vi "ReadI32Data.vi"(7 "無ければ作成(T)":bool=TRUE, 8 "Error In":errorcluster caption="エラー入力", 10 "データ":T2, 11 "refnum":T1) -> (0 "Error Out":errorcluster caption="エラー出力", 2 "数値":i32, 3 "refnum out":T1 caption="refnum出力")   [LabVIEW 2015]
doc: "iniファイルからI32データを読み込みます。"
uses:
  <vilib>/Utility/config.llb/Config Data RefNum.ctl
  <vilib>/Utility/config.llb/Read Key (I32).vi
  <vilib>/Utility/config.llb/Write Key (I32).vi
  <vilib>/Utility/config.llb/NI_LVConfig.lvlib
panel:
  # "■IniファイルからI32データを読込む"
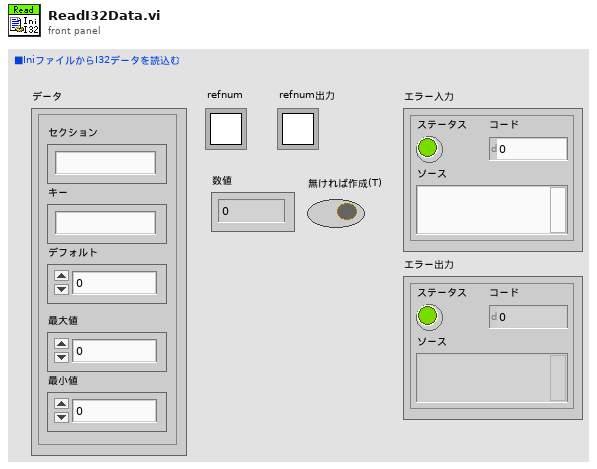
[diagram p1: front panel]
types:
  T1 = typedef "NI_LVConfig.lvlib/Config Data RefNum.ctl" = refnum<k1>
  T2 = cluster{"セクション":string, "キー":string, "デフォルト":i32, "最大値":i32, "最小値":i32}
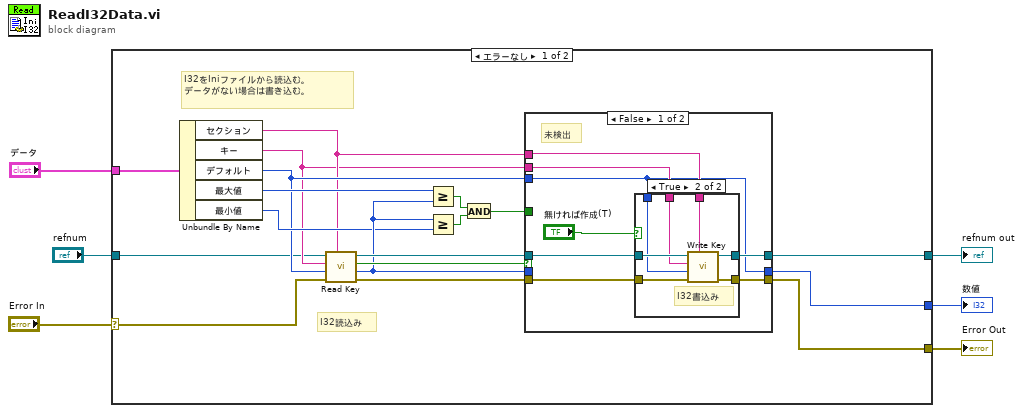
[diagram p0: block diagram]
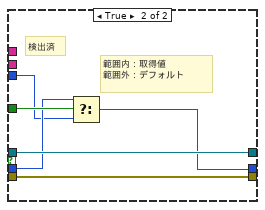
[diagram p3: hidden frame]
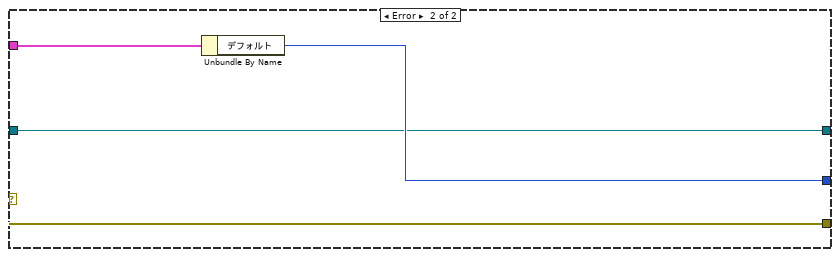
[diagram p4: hidden frame]
diagram:
  n1 = case shown="エラーなし" "Error In" {
    selector: "Error In" -> [w11 w51]
    tunnel: [w12 w51] -> w6
    tunnel: [w10 w49] -> w4
    tunnel: "データ" -> [w9 w50]
    tunnel: [w8 w48] -> w2
    tunnel: "refnum" -> [w7 w48]
    frame No Error {
      # "I32をIniファイルから読込む。\nデータがない場合は書き込む。"
      # "I32読込み"
      n2 = Unbundle By Name(w9) -> ("セクション"=w14:string, "キー"=w13:string, "デフォルト"=w15:i32, "最大値"=w21:i32, "最小値"=w19:i32)
      n3 = call-poly <vilib>:"Read Key.vi"("section"=w14, "error in (no error)"=w11, "default value"=w15, "key"=w13, "refnum"=w7) -> ("error out"=w22:errorcluster, "value"=w20:i32, "found?"=w24:bool, "refnum out"=w23:T1)  [unwired: 3 in]
      n4 = Greater Or Equal?(x=w21, y=w20) -> (x >= y?=w17:bool)
      n5 = Greater Or Equal?(x=w20, y=w19) -> (x >= y?=w18:bool)
      n6 = And(x=w17, y=w18) -> (x .and. y?=w16:bool)
      n7 = case shown="FALSE" w24 {
        tunnel: w23 -> [w32 w47]
        tunnel: [w31 w47] -> w8
        tunnel: w20 -> [_ w44]
        tunnel: [w26 w42] -> w10
        tunnel: w22 -> [w30 w46]
        tunnel: [w29 w46] -> w12
        tunnel: w16 -> [_ w45]
        tunnel: w15 -> [w26 w43]
        tunnel: w14 -> [w28 _]
        tunnel: w13 -> [w27 _]
        frame False {
          # "未検出"
          n8 = case shown="TRUE" "無ければ作成(T)" {
            tunnel: w32 -> [w34 w41]
            tunnel: [w34 w40] -> w31
            tunnel: w30 -> [w33 w39]
            tunnel: [w33 w38] -> w29
            tunnel: w28 -> [_ w37]
            tunnel: w27 -> [_ w36]
            tunnel: w26 -> [_ w35]
            frame False {
            }
            frame True {
              # "I32書込み"
              n9 = call-poly <vilib>:"Write Key.vi"("section"=w37, "error in (no error)"=w39, "value"=w35, "key"=w36, "refnum"=w41) -> ("error out"=w38:errorcluster, "refnum out"=w40:T1)  [unwired: 4 in, 1 out]
            }
          }
        }
        frame True {
          # "範囲内：取得値\n範囲外：デフォルト"
          # "検出済"
          n10 = Select(t=w44, s=w45, f=w43) -> (s? t:f=w42:i32)
        }
      }
    }
    frame Error {
      n11 = Unbundle By Name(w50) -> ("デフォルト"=w49:i32)
    }
  }
  "Error Out" <- w6
  "数値" <- w4
  "refnum out" <- w2
